vi "Cleanup.vi"(8 "error in (no error)":errorcluster, 11 "DeviceArrayPanel in":refnum<class "DeviceArrayPanel.lvclass">) -> (0 "error out":errorcluster)   [LabVIEW 2020, in "PicoG-App.lvlib" / "DeviceArrayPanel.lvclass"]
uses:
  DeviceArrayPanel.lvclass
  DeviceArrayPanel.lvclass/DeviceArrayPanel.ctl
  <vilib>/IlluminatedG/IG OOPanel/OOPanel/ArrayPanel/ArrayPanel.lvclass
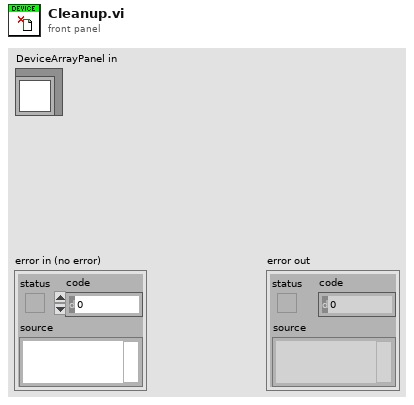
[diagram p1: front panel]
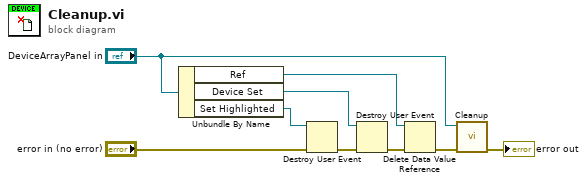
[diagram p0: block diagram]
diagram:
  n1 = Unbundle By Name("DeviceArrayPanel in") -> ("Ref"=w8:refnum<data-value>, "Device Set"=w9:refnum<user-event>, "Set Highlighted"=w2:refnum<user-event>)
  n2 = Destroy User Event(user event=w2, error in="error in (no error)") -> (error out=w3:errorcluster)
  n3 = Destroy User Event(user event=w9, error in=w3) -> (error out=w7:errorcluster)
  n4 = Delete Data Value Reference(data value reference=w8, error in=w7) -> (error out=w4:errorcluster)  [unwired: 1 out]
  n5 = call-parent "Cleanup.vi"("error in (no error)"=w4, "ArrayPanel in"="DeviceArrayPanel in") -> ("error out"=→"error out":errorcluster)  [unwired: 9 in]
